vi "UI_test.vi"() -> ()   [LabVIEW 2017]
panel:
  out "Waveform Chart 2":cluster{dbl, dbl, dbl}(graph)
  out "x":dbl
  out "y":dbl
  in  "stop":bool
  out "atan2(y,x)":dbl
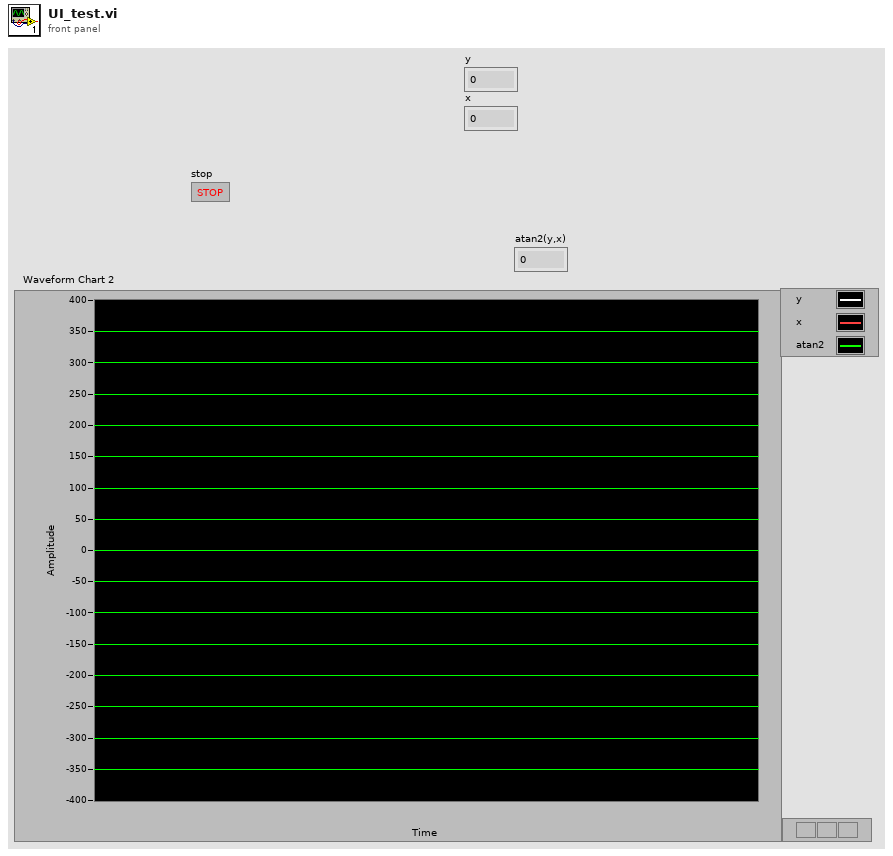
[diagram p1: front panel]
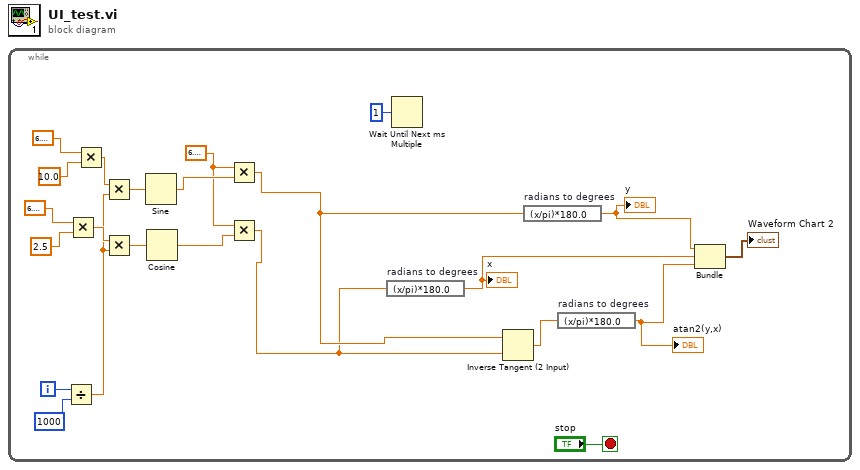
[diagram p0: block diagram]
diagram:
  n1 = while {
    i -> [w18]
    stop <- "stop" stop-if-true
    w11 = 6.283185307179586
    n2 = Divide(x=w18, y=1000) -> (x/y=w2:dbl)
    n3 = Multiply(x=6.283185307179586, y=2.5 ("x")) -> (x*y=w3:dbl)
    n4 = Multiply(x=6.283185307179586, y=10.0 ("x")) -> (x*y=w19:dbl)
    n5 = Multiply(x=w19, y=w2) -> (x*y=w15:dbl)
    n6 = Multiply(x=w3, y=w2) -> (x*y=w1:dbl)
    n7 = Sine(x=w15) -> (sin(x)=w16:dbl)
    n8 = Cosine(x=w1) -> (cos(x)=w10:dbl)
    n9 = Multiply(x=w11, y=w16) -> (x*y=w14:dbl)
    n10 = Multiply(x=w11, y=w10) -> (x*y=w9:dbl)
    n11 = expression code="(x/pi)*180.0" "radians to degrees"(w9) -> (w7:dbl)
    "x" <- w7
    n12 = Wait Until Next ms Multiple(millisecond multiple=u32 1) -> ()  [unwired: 1 out]
    n13 = Inverse Tangent (2 Input)(1:w9, 2:w14) -> (0:w13:dbl)
    n14 = expression code="(x/pi)*180.0" "radians to degrees"(w14) -> (w8:dbl)
    "y" <- w8
    n15 = expression code="(x/pi)*180.0" "radians to degrees"(w13) -> (w6:dbl)
    "atan2(y,x)" <- w6
    n16 = Bundle(w8, w7, w6) -> (→"Waveform Chart 2":cluster{dbl, dbl, dbl})  [unwired: 1 in]
  }
